vi "Compare Rects.vi"(8 "Bounding Rect":T1, 11 "Circle Rect":cluster{dbl, dbl, dbl, dbl}) -> (2 "Score":dbl)   [LabVIEW 2015]
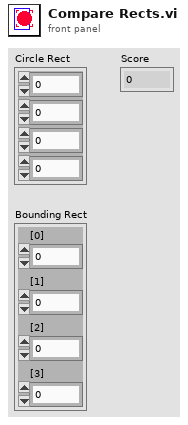
[diagram p1: front panel]
types:
  T1 = cluster{"[0]":dbl, "[1]":dbl, "[2]":dbl, "[3]":dbl}
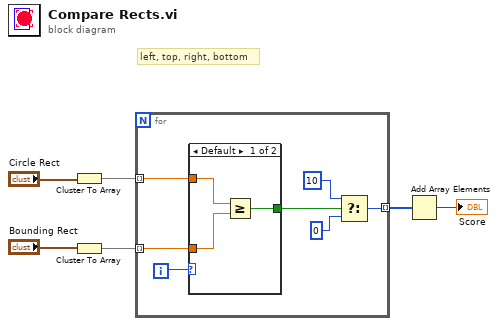
[diagram p0: block diagram]
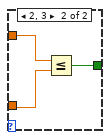
[diagram p2: hidden frame]
diagram:
  # "left, top, right, bottom"
  n1 = Cluster To Array(cluster="Circle Rect") -> (array=w4:dbl[])
  n2 = Cluster To Array(cluster="Bounding Rect") -> (array=w3:dbl[])
  n3 = for {
    tunnel: w4 -> [w12] mode=indexing
    tunnel: w3 -> [w11] mode=indexing
    tunnel: [w7] -> w2 mode=indexing
    i -> [w13]
    n4 = case shown="Default" w13 {
      tunnel: w12 -> [w16 w19]
      tunnel: w11 -> [w15 w18]
      tunnel: [w14 w17] -> w9
      frame Default {
        n5 = Greater Or Equal?(x=w16, y=w15) -> (x >= y?=w14:bool)
      }
      frame 2, 3 {
        n6 = Less Or Equal?(x=w19, y=w18) -> (x <= y?=w17:bool)
      }
    }
    n7 = Select(t=10, s=w9, f=0) -> (s? t:f=w7:i32)
  }
  n8 = Add Array Elements(numeric array=w2) -> (sum=→"Score":i32)
